vi "Unflatten From JSON String(lv-apt).vi"(6 "Nulls as Defaults (F)":bool, 7 "Type and Defaults":variant, 8 "error in (no error)":errorcluster, 11 "JSON String":string) -> (0 "error out":errorcluster, 3 "Variant":variant)   [LabVIEW 2019, in "lv-apt-json-file.lvlib"]
uses:
  lv-apt-json-file.lvlib
  <vilib>/addons/_JKI.lib/Serialization/JSON/JKI JSON Serialization.lvlib
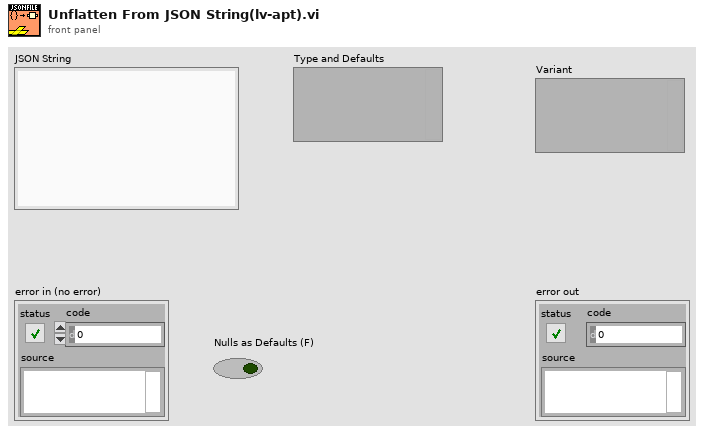
[diagram p1: front panel]
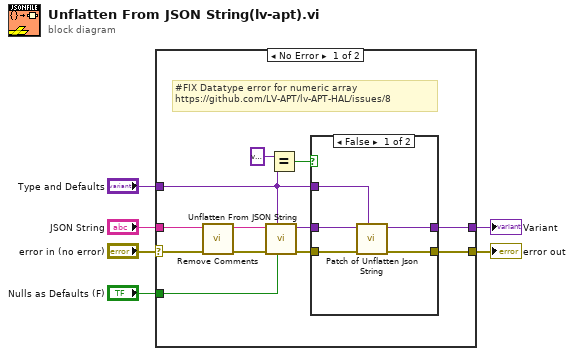
[diagram p0: block diagram]
diagram:
  n1 = case shown="No Error" "error in (no error)" {
    selector: "error in (no error)" -> [w8 w26]
    tunnel: "Nulls as Defaults (F)" -> [w18 _]
    tunnel: [w17 _] -> w5
    tunnel: "JSON String" -> [w16 _]
    tunnel: [w14 w26] -> w3
    tunnel: "Type and Defaults" -> [w12 _]
    frame No Error {
      # "#FIX Datatype error for numeric array\nhttps://github.com/LV-APT/lv-APT-HAL/issues/8"
      n2 = call "Remove Comments.vi"("error in (no error)"=w8, "String"=w16) -> ("error out"=w7:errorcluster, "string"=w9:string)  [unwired: 8 in]
      n3 = call <vilib>:"Unflatten From JSON String.vi"("Nulls as Defaults (F)"=w18, "Type and Defaults"=w12, "error in (no error)"=w7, "JSON String"=w9) -> ("error out"=w15:errorcluster, "Variant"=w13:variant)  [unwired: 6 in]
      n4 = Equal?(x=variant ("Type and Defaults"), y=w12) -> (x = y?=w11:bool)
      n5 = case shown="False" w11 {
        tunnel: [w23 w25] -> w17
        tunnel: w15 -> [w22 w24]
        tunnel: [w21 w24] -> w14
        tunnel: w12 -> [w20 _]
        tunnel: w13 -> [w19 w25]
        frame False {
          n6 = call "Patch of Unflatten Json String.vi"("VCluster"=w20, "error in (no error)"=w22, "Variant in"=w19) -> ("error out"=w21:errorcluster, "Variant out"=w23:variant)  [unwired: 7 in]
        }
        frame True {
        }
      }
    }
    frame Error {
    }
  }
  "Variant" <- w5
  "error out" <- w3
